vi "Curtin1_Acquire.vi"(8 "MainVI":refnum<vi>, 11 "Settings":T3={"Name of test"="ScratchPad", "Date"=timestamp(0 s since 1904-01-01), "Location"="Home", "Template"="ScratchPad", "Soundcard"="OCTA-CAPTURE", "resolution"=32, "Sampling rate"=48000, "Ch1 Gain "=25.0, "Ch2 Gain"=10.0, "Sample time (s)"=0.3, "Pre-trigger (s)"=0.001, "Hammer Threshold"=10.0, "Positions"=12, "Taps/Position"=5, "Set Names"="H,V", "Freq resolution"=1.0, "Hammer cutoff"=0.025, "Mic cutoff"=0.25, "Double bounce "=10.0, "Hammer Cal"=10.0, "dB Offset"=0.0, "Accel Cal"=10.0, "Vibrometer Cal"=0.0, "Mic Cal"=0.0, "Output"=2, "Voltage Cal"=0.01, "Vibrometer Port"="ASRL27::INSTR", "Range"=4, "High Pass"=2, "Bandwidth"=4, "X Range"=[], "Y Range"=[], "dB Spread"=0.0, "Trigger"=0, "Ch_1"=25, "Ch_2"=25, "flip?"=FALSE, "60Hz"=FALSE, "Time offset"=0.0, "Piezo Cal"=1.0, "Default Notes"="", "Tom"=FALSE} {"Ch_2" min=1 step=1; "Ch_1" min=1 max=100 step=1; "Trigger" items=["Hammer (force)", "Self-tap", "Spacebar"]; "Bandwidth" items=["1 kHz"=1, "5 kHz"=5, "10 kHz"=10, "25 kHz"=25, "50 kHz"=50, "100 kHz"=100]; "High Pass" items=["Off", "13 Hz", "104 Hz"]; "Range" items=["10 mm/s"=1, "20 mm/s"=2, "50 mm/s"=5, "100 mm/s"=10, "200 mm/s"=20, "500 mm/s"=50, "1 m/s"=100, "2 m/s"=200]; "Output" items=["Accelerometer", "Speed (from acceleration)", "Microphone", "Vibrometer", "Piezo"]; "Voltage Cal" format="%#_13g"; "Ch2 Gain" format="%#_13g"; "Ch1 Gain" format="%#_13g"; "Double bounce" min=0.0; "Mic cutoff" min=0.0 format="%#_4g"; "Hammer cutoff" min=0.0 format="%#_4g"; "Freq resolution" min=0.0; "Pre-trigger (s)" format="%#_13g"; "Date" format="%<%H:%M\n%d/%m/%y>T"; "resolution" items=["16 bit"=16, "24 bit"=24, "32 bit"=32]; "Sampling rate" items=["22050 samp/s"=22050, "44100 samp/s"=44100, "48000 samp/s"=48000]}) -> (1 "Name Change?":bool, 2 "Data?":bool, 3 "Average FRF":cluster{dbl, "df":dbl, dbl[]}[](graph))   [LabVIEW 2022 SP3]
uses:
  <extravilib>/ChannelInstances/Tag-a[.](wfm(dbl)).lvlib
  Mic/Mic_Global.vi
  <extravilib>/ChannelInstances/Lossy Stream-a[.](wfm(dbl)).lvlib
  AmpCtrl.ctl
  PreferencesControl.ctl
panel:
  in  "Record Button":bool=TRUE
  in  "Tab Control":enum32{"graphs", "settings", "Notes"}(tab)
  in  "AddPhoto":bool
  out "color":string
  in  "Move":bool
  in  "Motor Settings":bool
  in  "Tap":bool
  in  "Method":enum16{"Sqrt(H1H2)", "H1", "H2"}(ring)
  in  "History":bool=TRUE
  in  "Help":bool
  in  "Beam":bool
  in  "rescale Y Axes":bool
  in  "Open Sound":bool
  in  "View":u16(ring) items=["Raw", "Volts", "Units (Pa, N, etc)"]
  out "Hammer Spectrum":cluster{dbl, "df":dbl, "FFT {X}":dbl[]}[](graph)
  out "Hammer Data":cluster{dbl, "dt":dbl, "Y":dbl[]}[](graph)
  out "Microphone Data":cluster{dbl, "dt":dbl, "Y":dbl[]}[](graph)
  out "Volume":T1 {"Mic" scale=0.0..100.0; "Hammer" scale=0.0..100.0}
  in  "OpenVibrometer":bool
  in  "New":bool
  in  "Save SP":bool
  in  "Export":bool
  in  "Plot View":T2={"Alerts"=FALSE, "Log X Axis"=TRUE, "dB scale"=TRUE, "Averaging"=TRUE, "Fade"=0.0, "Centroids?"=FALSE, "line thickness"=1}
  in  "Locked":bool
  in  "Notes":string
  in  "Done":bool
  out "Progress Bar":picture
  in  "zoom":bool
  in  "dB Spread":dbl=40.0
  in  "rescale Y":bool
  in  "stop":bool
  out "Alarms":string
  in  "Colors":u16(ring) items=["24 Colors", "rear"]
  # "Hz"
  # "dB"
  # "dB"
  # "sec"
  # "sec"
  # "mV/Pa"
  # "mV/m/s2"
  # "mV/mm/s"
  # "V/N"
  # "sec"
  # "sec"
  # "mV/N"
  # "%"
  # "%"
  # "sec"
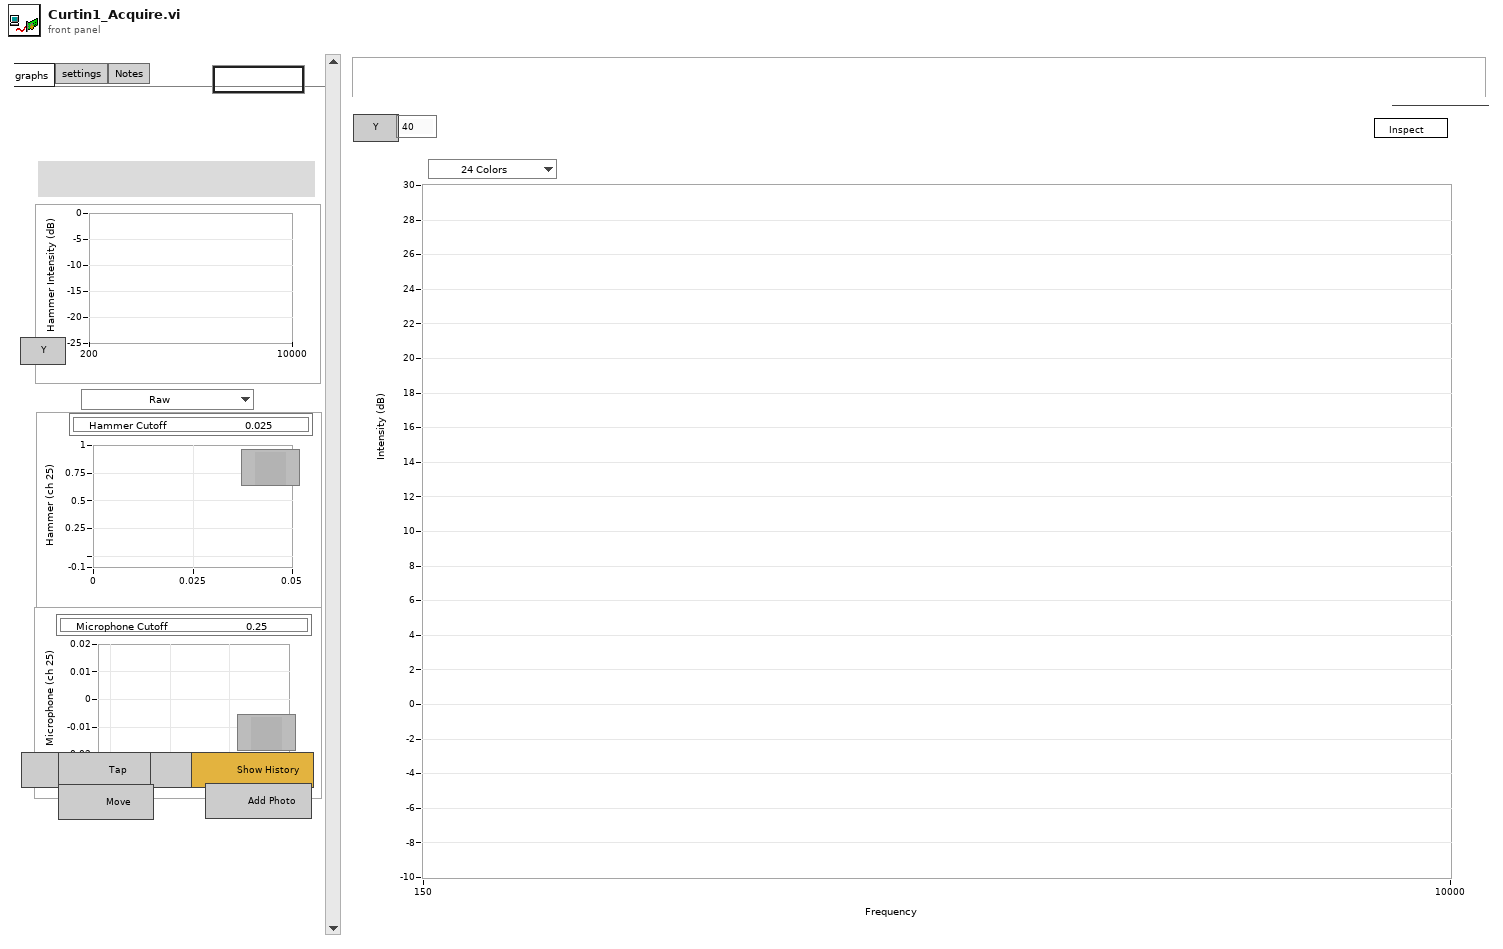
[diagram p1: front panel]
types:
  T1 = typedef "AmpCtrl.ctl" = cluster{"Hammer":u8, "Mic":u8, "Mic In":string}
  T2 = cluster{"Alerts":bool, "Log X Axis":bool, "dB scale":bool, "Averaging":bool, "Fade":dbl, "Centroids?":bool, "line thickness":u8}
  T3 = typedef "PreferencesControl.ctl" = cluster{"Name of test":string, "Date":timestamp, "Location":string, "Template":string, "Soundcard":string, "resolution":u16, "Sampling rate":u16, "Ch1 Gain ":dbl, "Ch2 Gain":dbl, "Sample time (s)":dbl, "Pre-trigger (s)":dbl, "Hammer Threshold":dbl, "Positions":i16, "Taps/Position":i16, "Set Names":string, "Freq resolution":dbl, "Hammer cutoff":dbl, "Mic cutoff":dbl, "Double bounce ":dbl, "Hammer Cal":dbl, "dB Offset":dbl, "Accel Cal":dbl, "Vibrometer Cal":dbl, "Mic Cal":dbl, "Output":u16, "Voltage Cal":dbl, "Vibrometer Port":refnum<visa-resource-name>, "Range":u16, "High Pass":u16, "Bandwidth":u16, "X Range":cluster{"Minimum":dbl, "Maximum":dbl, "Increment":dbl, "Minor Increment":dbl, "Start":dbl}[], "Y Range":cluster{"Minimum":dbl, "Maximum":dbl, "Increment":dbl, "Minor Increment":dbl, "Start":dbl}[], "dB Spread":dbl, "Trigger":u16, "Ch_1":u8, "Ch_2":u8, "flip?":bool, "60Hz":bool, "Time offset":dbl, "Piezo Cal":dbl, "Default Notes":string, "Tom":bool}
  T4 = enum32{"Invalid", "Standard", "Closed", "Hidden", "Minimized", "Maximized"}
  T5 = enum16{"Initialize", "Free run", "One Shot - waiting", "One Shot - triggered", "Wait", "Close"}
  T6 = enum16{"Always On", "Always Off", "Off While Running"}
  T7 = enum8{"Enabled", "Disabled", "Disabled and Grayed Out"}
  T8 = typedef "Tag-a[.](wfm(dbl)).lvlib/))Channel.ctl" = refnum<queue>
  T9 = typedef "Lossy Stream-a[.](wfm(dbl)).lvlib/)Channel.ctl" = refnum<queue>
  T10 = typedef "LVBoundsTypeDef.ctl" = cluster{"Width":u32, "Height":u32}
  T11 = cluster{"Minimum":dbl, "Maximum":dbl, "Increment":dbl, "Minor Increment":dbl, "Start":dbl}
  T12 = typedef "eventvkey.ctl" = enum16{"ASCII", "Enter", "Return", "Shift", "Ctrl", "Alt", "Cmd", "Opt", "Caps", "NumLock", "Clear", "Break", "Up", "Down", "Left", "Right", "Insert", "Delete", "Home", "End", "PageUp", "PageDown", "Escape", "Help", "Pause", "ScrollLock", "F1", "F2", "F3", "F4", "F5", "F6", "F7", "F8", "F9", "F10", "F11", "F12", "F13", "F14", "F15", "F16", "F17", "F18", "F19", "F20", "F21", "F22", "F23", "F24", "Play", "VolumeUp", "VolumeDown", "Mute", "Two Byte Char"}
  T13 = typedef "LVMouseTypeDef.ctl" = cluster{"Mouse Position":cluster{"X":i32, "Y":i32}, "Mouse Modifiers":cluster{"Button Down":bool, "Shift Mod":bool, "Menu Mod":bool, "Option Mod":bool}}
  T14 = typedef "LVRangeTypeDef.ctl" = cluster{"Minimum":dbl, "Maximum":dbl, "Increment":dbl, "Minor Increment":dbl, "Start":dbl}
  T15 = cluster{"Minimum":dbl, "Maximum":dbl, "Increment":dbl, "Minor Increment":dbl, "Start":dbl}[]
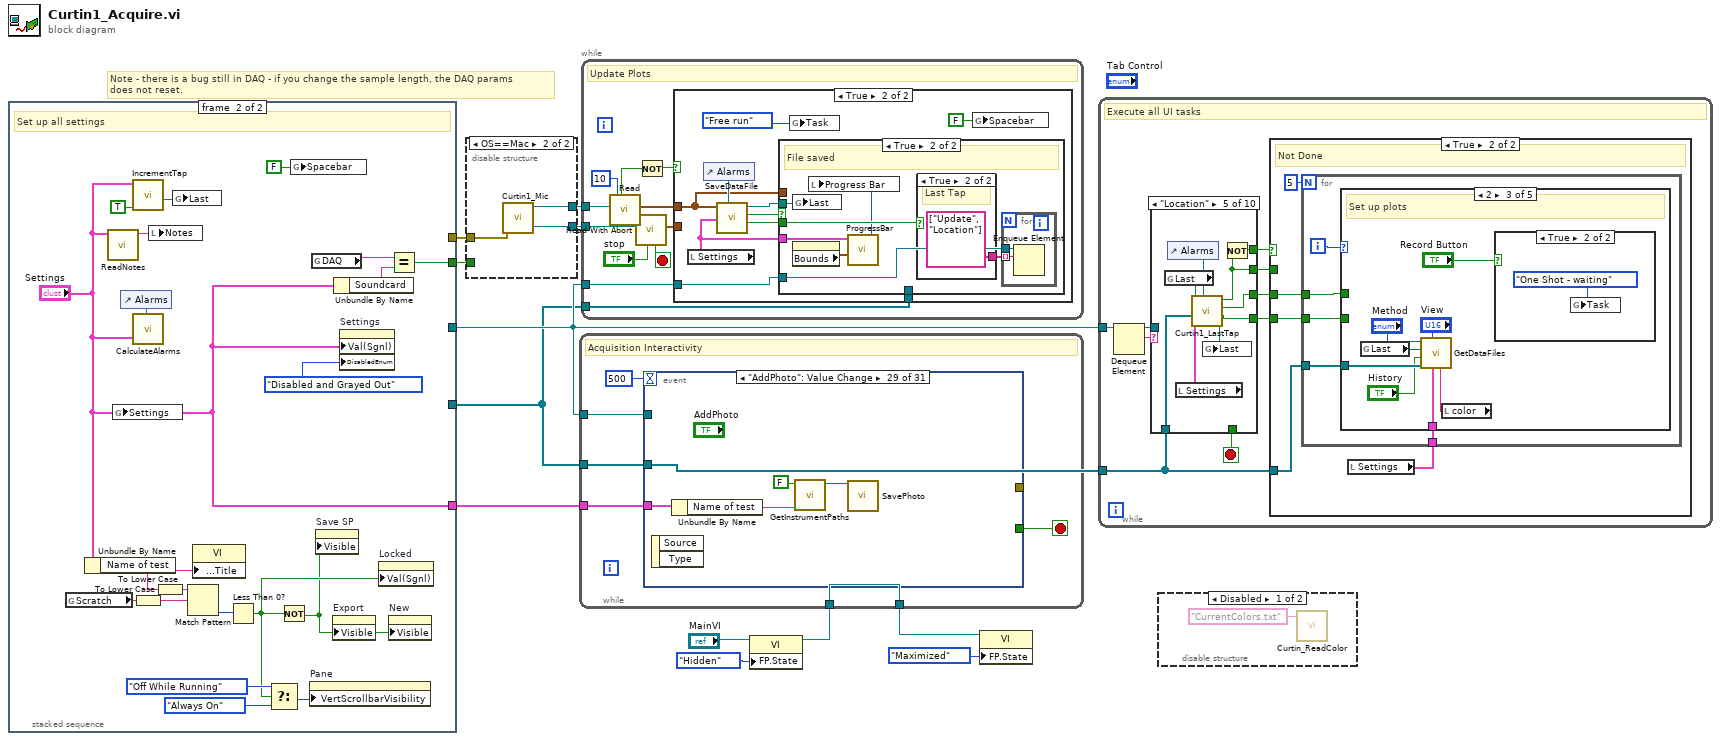
[diagram p0: block diagram]
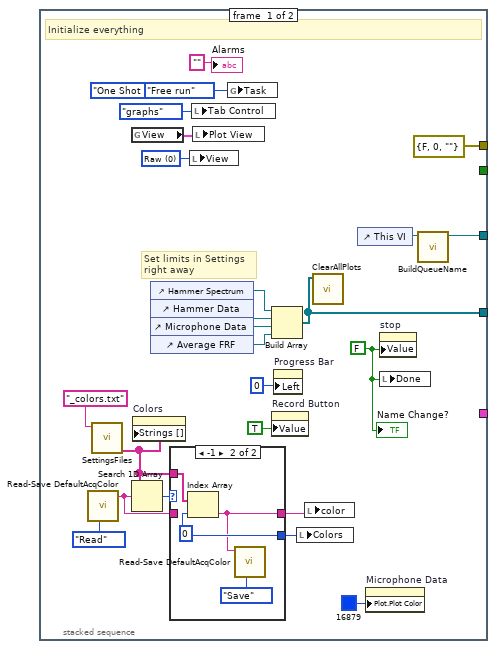
[diagram p3: hidden frame]
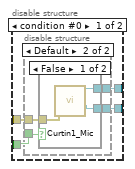
[diagram p5: hidden frame]
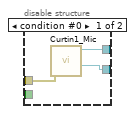
[diagram p6: hidden frame]
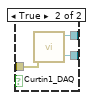
[diagram p7: hidden frame]
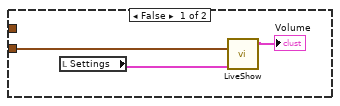
[diagram p8: hidden frame]
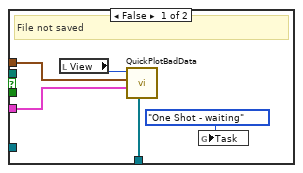
[diagram p9: hidden frame]
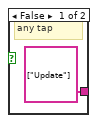
[diagram p10: hidden frame]
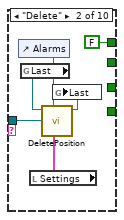
[diagram p12: hidden frame]
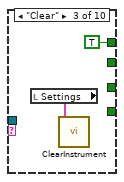
[diagram p13: hidden frame]
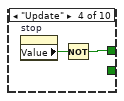
[diagram p14: hidden frame]
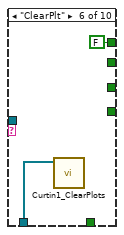
[diagram p15: hidden frame]
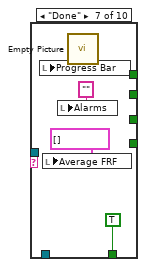
[diagram p16: hidden frame]
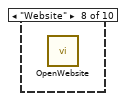
[diagram p17: hidden frame]
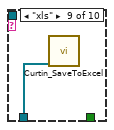
[diagram p18: hidden frame]
diagram:
  # "Note - there is a bug still in DAQ - if you change the sample length, the DAQ params \ndoes not reset."
  n1 = stacked-sequence {
    tunnel: [_ "Settings"] -> w5
    tunnel: [_ w52] -> w4
    tunnel: [w26 _] -> w3
    tunnel: [errorcluster {"status"=FALSE, "code"=0, "source"=""} ("error in (no error)") _] -> w2
    tunnel: [w20 _] -> w1
    frame #0 {
      w33 = u16 0 items=["Raw", "Volts", "Units (Pa, N, etc)"] ("View")
      w35 = FALSE ("stop")
      # "Set limits in Settings \nright away"
      # "Initialize everything"
      n2 = call "Read-Save DefaultAcqColor.vi"("Task"=enum16{"Save", "Read"}."Read") -> ("palette name Out"=w13:string)  [unwired: 9 in, 1 out]
      n3 = call "SettingsFiles.vi"("settings file name"="_colors.txt" ("pattern")) -> ("filenames"=w14:string[])  [unwired: 9 in, 1 out]
      n4 = global read "Mic_Global.vi" "View"() -> (w36:T2)
      n5 = Search 1D Array(1D array=w14, element=w13) -> (index of element=w15:i32)  [unwired: 1 in]
      n6 = property on="Colors" class="Ring (strict)"("Strings []"=w14) -> ()  [unwired: 2 in, 2 out]
      n7 = control-ref of="Hammer Spectrum"() -> (w21:refnum<vi>)
      n8 = control-ref of="Hammer Data"() -> (w22:refnum<vi>)
      n9 = control-ref of="Microphone Data"() -> (w23:refnum<vi>)
      n10 = control-ref of="Average FRF"() -> (w24:refnum<vi>)
      n11 = case shown="-1" w15 {
        selector: w15 -> [w38 _]
        tunnel: [w38 w43] -> w18
        tunnel: [w39 w40] -> w17
        tunnel: w14 -> [_ w42]
        tunnel: w13 -> [w39 _]
        frame Default {
        }
        frame -1 {
          w43 = 0
          n12 = Index Array(array=w42, index=w43) -> (element=w40:string)
          n13 = call "Read-Save DefaultAcqColor.vi"("Task"=enum16{"Save", "Read"}."Save", "acq color palette"=w40) -> ()  [unwired: 8 in, 2 out]
        }
      }
      n14 = local write "View"(w33) -> ()
      n15 = local write "Tab Control"(enum32{"graphs", "settings"}."graphs" ("Tab Control")) -> ()
      n16 = local write "Plot View"(w36) -> ()
      n17 = global write "Mic_Global.vi" "Task"(T5."One Shot - waiting" ("Task")) -> ()
      n18 = global write "Mic_Global.vi" "Task"(T5."Free run" ("Task")) -> ()
      n19 = Build Array(w21, w22, w23, w24) -> (w20:refnum<vi>[])
      n20 = property on="Record Button" class="Bool (strict)"("Value"=TRUE ("Good point?")) -> ()  [unwired: 2 in, 2 out]
      n21 = property on="Progress Bar" class="Pict"("Left"=i16 0 ("Origin:Left")) -> ()  [unwired: 2 in, 2 out]
      n22 = local write "Colors"(w18) -> ()
      n23 = local write "color"(w17) -> ()
      n24 = call "ClearAllPlots.vi"("Array"=w20) -> ()  [unwired: 11 in]
      n25 = control-ref of="This VI"() -> (w27:refnum<vi>)
      n26 = property on="Microphone Data" class="WFGraph (strict)"("Plot.Plot Color"=u32 16879) -> ()  [unwired: 2 in, 2 out]
      n27 = property on="stop" class="Bool (strict)"("Value"=w35) -> ()  [unwired: 2 in, 2 out]
      n28 = local write "Done"(w35) -> ()
      n29 = call "BuildQueueName.vi"("VI in"=w27) -> ("Queue out"=w26:refnum<queue>)  [unwired: 9 in, 1 out]
      "Name Change?" <- w35
      "Alarms" <- "" ("Alarms")
    }
    frame #1 {
      # "Set up all settings"
      n30 = global read "Mic_Global.vi" "Scratch"() -> (w58:string)
      n31 = Unbundle By Name("Settings") -> ("Name of test"=w57:string)
      n32 = call "ReadNotes.vi"("Settings"="Settings") -> ("Notes"=w62:string)  [unwired: 9 in, 1 out]
      n33 = global write "Mic_Global.vi" "Settings"("Settings") -> ()
      n34 = control-ref of="Alarms"() -> (w59:refnum<vi>)
      n35 = call "IncrementTap.vi"("Reset?"=TRUE, "Settings"="Settings") -> ("Last Data Set"=w61:path)  [unwired: 4 in, 5 out]
      n36 = call "CalculateAlarms.vi"("Settings"="Settings", "Alarm"=w59) -> ()  [unwired: 8 in, 2 out]
      n37 = To Lower Case(string=w58) -> (all lower case string=w45:string)
      n38 = local write "Notes"(w62) -> ()
      n39 = To Lower Case(string=w57) -> (all lower case string=w46:string)
      n40 = global write "Mic_Global.vi" "Last"(w61) -> ()
      n41 = Match Pattern(string=w46, regular expression=w45) -> (offset past match=w56:i32)  [unwired: 1 in, 3 out]
      n42 = property class="VI"("Front Panel.Title"=w57) -> ()  [unwired: 2 in, 2 out]
      n43 = Less Than 0?(x=w56) -> (x < 0?=w48:bool)
      n44 = Select(t=T6."Off While Running" ("Vertical Scrollbar Visibility"), s=w48, f=T6."Always On" ("Vertical Scrollbar Visibility")) -> (s? t:f=w55:T6)
      n45 = Not(x=w48) -> (.not. x?=w47:bool)
      n46 = global write "Mic_Global.vi" "Spacebar"(FALSE ("Spacebar")) -> ()
      n47 = property on="Pane" class="Pane"("VertScrollbarVisibility"=w55) -> ()  [unwired: 2 in, 2 out]
      n48 = global read "Mic_Global.vi" "DAQ"() -> (w54:string)
      n49 = property on="Save SP" class="Bool"("Visible"=w47) -> ()  [unwired: 2 in, 2 out]
      n50 = property on="Export" class="Bool"("Visible"=w47) -> ()  [unwired: 2 in, 2 out]
      n51 = Unbundle By Name("Settings") -> ("Soundcard"=w53:string)
      n52 = property on="Settings" class="Clust (strict)"("Val(Sgnl)"="Settings", "DisabledEnum"=T7."Disabled and Grayed Out" ("Disabled")) -> ()  [unwired: 2 in, 2 out]
      n53 = property on="Locked" class="Bool (strict)"("Val(Sgnl)"=w48) -> ()  [unwired: 2 in, 2 out]
      n54 = Equal?(x=w54, y=w53) -> (x = y?=w52:bool)
      n55 = property on="New" class="Bool"("Visible"=w47) -> ()  [unwired: 2 in, 2 out]
    }
  }
  n56 = disable-structure shown="OS==Mac" {
    disable-tunnel: w2 -> [w67 w83]
    disable-tunnel: [w66 w81] -> w12
    disable-tunnel: [w65 w82] -> w11
    disable-tunnel: w4 -> [w64 _]
    frame condition #0 {
      n57 = disable-structure shown="Default" {
        disable-tunnel: w67 -> [w68 w72]
        disable-tunnel: [w70 w74] -> w66
        disable-tunnel: [w69 w73] -> w65
        disable-tunnel: w64 -> [_ w71]
        frame condition #0 {
          n58 = call "Curtin1_Mic.vi"("error in (no error)"=w68) -> ("latest data"=w70:T8, "Tap"=w69:T9)  [unwired: 9 in]
        }
        frame condition #1 (active) {
          n59 = case shown="False" w71 {
            tunnel: [w76 w80] -> w74
            tunnel: [w75 w79] -> w73
            tunnel: w72 -> [w77 w78]
            frame False {
              n60 = call "Curtin1_Mic.vi"("error in (no error)"=w77) -> ("latest data"=w76:T8, "Tap"=w75:T9)  [unwired: 9 in]
            }
            frame True {
              n61 = call "Curtin1_DAQ.vi"("error in (no error)"=w78) -> ("Buffer"=w80:T8, "Tap"=w79:T9)  [unwired: 9 in]
            }
          }
        }
      }
    }
    frame condition #1 (active) {
      n62 = call "Curtin1_Mic.vi"("error in (no error)"=w83) -> ("latest data"=w81:T8, "Tap"=w82:T9)  [unwired: 9 in]
    }
  }
  n63 = while {
    tunnel: w11 -> [w94]
    tunnel: w12 -> [w91]
    tunnel: w3 -> [w85]
    tunnel: w1 -> [w84]
    stop <- w90 stop-if-true
    # "Update Plots"
    n64 = call <extravilib>:"Read.vi"("channel"=w94, "timeout in ms (-1)"=10) -> ("element"=w93:waveform(dbl)[], "timed out?"=w87:bool)  [unwired: 4 in, 4 out]
    n65 = call <extravilib>:"Read With Abort.vi"("abort"="stop", "channel"=w91) -> ("element"=w89:waveform(dbl)[], "aborted?"=w90:bool)  [unwired: 7 in, 1 out]
    n66 = Not(x=w87) -> (.not. x?=w86:bool)
    n67 = case shown="True" w86 {
      tunnel: w93 -> [_ w100]
      tunnel: w89 -> [w96 _]
      tunnel: w85 -> [_ w105]
      tunnel: w84 -> [_ w99]
      frame False {
        n68 = local read "Settings"() -> (w95:T3)
        n69 = call "LiveShow.vi"("Settings"=w95, "Buffer"=w96) -> ("Volume"=→"Volume":T1)  [unwired: 9 in]
      }
      frame True {
        n70 = local read "Settings"() -> (w101:T3)
        n71 = control-ref of="Alarms"() -> (w104:refnum<vi>)
        n72 = call "SaveDataFile.vi"("Settings"=w101, "Alarms"=w104, "Data"=w100) -> ("last tap?"=w106:bool, "New File?"=w107:bool, "new path"=w103:path)  [unwired: 4 in, 2 out]
        n73 = case shown="True" w107 {
          tunnel: w106 -> [_ w119]
          tunnel: w105 -> [_ w113]
          tunnel: w103 -> [_ w118]
          tunnel: w101 -> [w108 w116]
          tunnel: w100 -> [w109 _]
          tunnel: w99 -> [w110 _]
          frame False {
            # "File not saved"
            n74 = local read "View"() -> (w111:u16)
            n75 = call "QuickPlotBadData.vi"("Array"=w110, "Settings"=w108, "Data"=w109, "View"=w111) -> ()  [unwired: 8 in]
            n76 = global write "Mic_Global.vi" "Task"(T5."One Shot - waiting" ("Task")) -> ()
          }
          frame True {
            # "File saved"
            n77 = global write "Mic_Global.vi" "Last"(w118) -> ()
            n78 = property on="Progress Bar" class="Pict"() -> ("Bounds"=w114:T10)  [unwired: 2 in, 2 out]
            n79 = call "ProgressBar.vi"("Bounds"=w114, "Settings"=w116) -> ("Progress Bar"=w115:picture)  [unwired: 7 in, 2 out]
            n80 = local write "Progress Bar"(w115) -> ()
            n81 = case shown="True" w119 {
              tunnel: [string[] ["Update"] string[] ["Update", "Location"]] -> w117
              frame False {
                # "any tap"
              }
              frame True {
                # "Last Tap"
              }
            }
            n82 = for {
              tunnel: w117 -> [w121] mode=indexing
              tunnel: w113 -> [w120]
              n83 = Enqueue Element(queue=w120, element=w121) -> ()  [unwired: 2 in, 3 out]
            }
          }
        }
        n84 = global write "Mic_Global.vi" "Task"(T5."Free run" ("Task")) -> ()
        n85 = global write "Mic_Global.vi" "Spacebar"(FALSE ("Spacebar")) -> ()
      }
    }
  }
  n86 = property class="VI"(reference="MainVI", "FP.State"=T4."Hidden" ("Front Panel Window:State")) -> (reference out=w6:refnum<vi>)  [unwired: 1 in, 1 out]
  n87 = while {
    tunnel: w1 -> [w129]
    tunnel: w3 -> [w126]
    tunnel: [w125] -> w7
    tunnel: w6 -> [w125]
    tunnel: w5 -> [w124]
    stop <- w127 stop-if-true
    # "Acquisition Interactivity"
    n88 = event shown="[28] \"AddPhoto\": Value Change" {
      selector: _ -> [_ _ _ _ _ _ _ _ _ _ _ _ _ _ _ _ _ _ _ _ _ _ _ _ _ _ _ _ _ _ _]
      dyn-events: _ -> [_ _ _ _ _ _ _ _ _ _ _ _ _ _ _ _ _ _ _ _ _ _ _ _ _ _ _ _ _ _ _]
      timeout: 500 -> [_ _ _ _ _ _ _ _ _ _ _ _ _ _ _ _ _ _ _ _ _ _ _ _ _ _ _ _ _ _ _]
      tunnel: [_ _ _ _ _ _ _ _ _ _ _ _ _ _ _ _ _ _ _ w263 _ _ _ _ _ _ _ _ _ _ w304] -> w127
      tunnel: w129 -> [w133 w145 _ _ _ w164 _ _ _ _ _ _ _ w209 _ _ _ _ _ _ _ _ _ _ _ _ _ _ _ _ _]
      tunnel: w126 -> [_ _ _ _ _ w168 _ w174 w179 w193 w200 w203 _ w208 _ _ _ _ _ w262 _ w278 _ _ _ _ _ _ _ _ w303]
      tunnel: [_ _ _ _ _ _ _ _ _ _ _ _ _ _ _ _ _ _ w248 _ _ _ _ _ _ w289 w295 _ _ _ _] -> _
      tunnel: w124 -> [_ _ _ _ _ _ _ _ _ _ _ _ _ _ _ _ w238 _ _ w258 _ _ _ w285 _ w288 _ _ w300 _ _]
      event "Hammer Data", "Microphone Data", "Average FRF", "Hammer Spectrum": Mouse Up {
        n89 = event-data() -> ("PlatMods.Shift"=w134:bool, "CtlRef"=w132:refnum<vi>)  [unwired: 1 in]
        n90 = local read "History"() -> (w136:bool)
        n91 = Search 1D Array(1D array=w133, element=w132) -> (index of element=w131:i32)  [unwired: 1 in]
        n92 = case shown="1, 2" w131 {
          tunnel: [9 0] -> w130
          frame 1, 2 {
          }
          frame Default {
          }
        }
        n93 = call "BuildZoomNames.vi"("History"=w136, "WaveformGraph in"=w132) -> ("Names"=w135:string[])  [unwired: 9 in]
        n94 = case shown="True" w134 {
          tunnel: w132 -> [_ w142]
          tunnel: w135 -> [_ w140]
          tunnel: w130 -> [_ w139]
          frame False {
          }
          frame True {
            n95 = local read "dB Spread"() -> (w141:dbl)
            n96 = call "GraphZoom.vi"("Plot"=w139, "Names"=w140, "dB Range"=w141, "Graph"=w142) -> ()  [unwired: 8 in]
          }
        }
      }
      event "zoom": Value Change {
        n97 = event-data() -> ()  [unwired: 1 in, 1 out]
        n98 = Index Array(array=w145, index=3) -> (element=w143:refnum<vi>)
        n99 = local read "History"() -> (w148:bool)
        n100 = call "BuildZoomNames.vi"("History"=w148, "WaveformGraph in"=w143) -> ("Names"=w147:string[])  [unwired: 9 in]
        n101 = local read "dB Spread"() -> (w146:dbl)
        n102 = call "GraphZoom.vi"("Names"=w147, "dB Range"=w146, "Graph"=w143) -> ()  [unwired: 9 in]
      }
      event "Microphone Data": Cursor Move {
        n103 = event-data() -> ("CursLoc.X"=w149:dbl)  [unwired: 1 in]
        n104 = property on="Mic cutoff" class="DigNum (strict)"("Val(Sgnl)"=w149) -> ()  [unwired: 2 in, 2 out]
      }
      event "Hammer Data": Cursor Move {
        n105 = event-data() -> ("CursIdx"=w151:i32, "CursLoc.X"=w152:dbl, "CursLoc.Y"=w150:dbl)  [unwired: 1 in]
        n106 = case shown="0" w151 {
          tunnel: w152 -> [w153 _]
          tunnel: w150 -> [_ w154]
          frame 0 {
            n107 = property on="Hammer cutoff" class="DigNum (strict)"("Val(Sgnl)"=w153) -> ()  [unwired: 2 in, 2 out]
          }
          frame Default {
            n108 = property on="Hammer Threshold" class="DigNum (strict)"("Val(Sgnl)"=w154) -> ()  [unwired: 2 in, 2 out]
          }
        }
      }
      event "Notes": Value Change {
        n109 = event-data() -> ()  [unwired: 1 in, 1 out]
        n110 = local read "Settings"() -> (w156:T3)
        n111 = call "Curtin1_SaveNotesFile.vi"("Notes"="Notes", "Settings in"=w156) -> ()  [unwired: 10 in]
      }
      event Value Change {
        n112 = event-data() -> ("NewVal"=w162:T3, "OldVal"=w161:T3)  [unwired: 1 in]
        n113 = Enqueue Element(queue=w168, element="Update") -> ()  [unwired: 2 in, 3 out]
        n114 = call "VibrometerSettings.vi"("OldVal"=w161, "NewVal"=w162) -> ("Settings"=w157:T3)  [unwired: 5 in, 4 out]
        n115 = global write "Mic_Global.vi" "Settings"(w157) -> ()
        n116 = call "Curtin1_SaveLastSettingsFile.vi"("Settings in"=w157) -> ()  [unwired: 11 in]
        n117 = call "Curtin1_updatePlots.vi"("plots"=w164, "Settings"=w157) -> ()  [unwired: 10 in]
        n118 = Unbundle By Name(w157) -> ("dB Spread"=w163:dbl, "Output"=w159:u16)
        n119 = call "Read_Write_Test_Parameters.vi"("Task"=enum16{"Save", "Read", "Clear"}."Save", "Settings"=w157) -> ("Settings"=w165:T3)  [unwired: 8 in, 1 out]
        n120 = local write "dB Spread"(w163) -> ()
        n121 = call "IncrementTap.vi"("Settings"=w165) -> ("Last Data Set"=w166:path)  [unwired: 5 in, 5 out]
        n122 = Equal?(x=u16 3 ("Output"), y=w159) -> (x = y?=w158:bool)
        n123 = global write "Mic_Global.vi" "Last"(w166) -> ()
        n124 = property on="Beam" class="Bool (strict)"("Visible"=w158) -> ()  [unwired: 2 in, 2 out]
      }
      event "dB Spread": Value Change {
        n125 = event-data() -> ("NewVal"=w171:dbl)  [unwired: 1 in]
        n126 = local read "Settings"() -> (w172:T3)
        n127 = Bundle By Name(cluster=w172, "dB Spread"=w171) -> (w170:T3)
        n128 = local write "Settings"(w170) -> ()
        n129 = global write "Mic_Global.vi" "Settings"(w170) -> ()
      }
      event Key Up {
        n130 = event-data() -> ("ScanCode"=w176:i16, "PlatMods.Shift"=w175:bool)  [unwired: 1 in]
        n131 = call "Check KeyUp.vi"("Shift"=w175, "ScanCode"=w176) -> ("Task"=w173:string)  [unwired: 9 in]
        n132 = case shown="Default" w173 {
          selector: w173 -> [_ w177]
          tunnel: w174 -> [_ w178]
          frame "" {
          }
          frame Default {
            n133 = Enqueue Element(queue=w178, element=w177) -> ()  [unwired: 2 in, 3 out]
          }
        }
      }
      event Key Down {
        n134 = event-data() -> ("VKey"=w180:T12)  [unwired: 1 in, 3 out]
        n135 = case shown="\"Up\", \"Down\"" w180 {
          selector: w180 -> [_ w184 w188]
          tunnel: w179 -> [_ w181 w186]
          frame "ASCII", Default {
          }
          frame "Left", "Right" {
            n136 = Format Into String(w184) -> (resulting string=w183:string)  [unwired: 3 in, 1 out]
            n137 = Enqueue Element(queue=w181, element="Update") -> ()  [unwired: 2 in, 3 out]
            n138 = call "FadeLeftRight.vi"("Key"=w183) -> ()  [unwired: 11 in]
          }
          frame "Up", "Down" {
            n139 = Format Into String(w188) -> (resulting string=w185:string)  [unwired: 3 in, 1 out]
            n140 = Enqueue Element(queue=w186, element="Update") -> ()  [unwired: 2 in, 3 out]
            n141 = call "ThicknessUpDown.vi"("Key"=w185) -> ()  [unwired: 11 in]
          }
        }
      }
      event "Progress Bar": Mouse Up {
        # "need to end free run\nif in Done condition"
        n142 = event-data() -> ()  [unwired: 1 in, 1 out]
        n143 = property on="Progress Bar" class="Pict"() -> ("Mouse"=w194:T13, "Bounds"=w192:T10)  [unwired: 2 in, 2 out]
        n144 = local read "Settings"() -> (w191:T3)
        n145 = global write "Mic_Global.vi" "Task"(T5."Free run" ("Task")) -> ()
        n146 = call "DetermineSetChosen.vi"("Settings"=w191, "Bounds"=w192, "Mouse"=w194) -> ("Queue Task"=w189:string)  [unwired: 7 in, 1 out]
        n147 = case shown="Default" w189 {
          selector: w189 -> [_ w195]
          tunnel: w193 -> [_ w198]
          tunnel: w191 -> [_ w197]
          frame "" {
          }
          frame Default {
            n148 = Enqueue Element(queue=w198, element=w195) -> ()  [unwired: 2 in, 3 out]
            n149 = control-ref of="Alarms"() -> (w196:refnum<vi>)
            n150 = call "CalculateAlarms.vi"("Settings"=w197, "Alarm"=w196) -> ()  [unwired: 8 in, 2 out]
          }
        }
      }
      event "Plot View": Value Change {
        n151 = event-data() -> ()  [unwired: 1 in, 4 out]
        n152 = Enqueue Element(queue=w200, element="Update") -> ()  [unwired: 2 in, 3 out]
        n153 = global write "Mic_Global.vi" "View"("Plot View") -> ()
      }
      event "View", "History", "Method": Value Change {
        n154 = event-data() -> ()  [unwired: 1 in, 4 out]
        n155 = Enqueue Element(queue=w203, element="Update") -> ()  [unwired: 2 in, 3 out]
      }
      event "Record Button": Value Change {
        n156 = event-data() -> ("NewVal"=w204:bool)  [unwired: 1 in]
        n157 = Select(t=T5."One Shot - waiting" ("Task"), s=w204, f=T5."Free run" ("Task")) -> (s? t:f=w206:T5)
        n158 = global write "Mic_Global.vi" "Task"(w206) -> ()
      }
      event "Average FRF", "Hammer Spectrum", "Microphone Data", "Hammer Data": Scale Range Change; "rescale Y": Value Change {
        n159 = event-data() -> ()  [unwired: 1 in, 1 out]
        n160 = stacked-sequence {
          tunnel: w209 -> [w211 w222 _]
          tunnel: w208 -> [_ _ w223]
          frame #0 {
            n161 = case shown="False" "rescale Y" {
              tunnel: w211 -> [_ w217]
              tunnel: "dB Spread" -> [_ w214]
              frame False {
              }
              frame True {
                n162 = Index Array(array=w217, index=3) -> (element=w215:refnum<vi>)
                n163 = call "AutoscaleYaxis.vi"("Has Coherence in plot?"=TRUE, "dB Range"=w214, "WaveformGraph in"=w215) -> ()  [unwired: 9 in]
              }
            }
          }
          frame #1 {
            n164 = call "GetPlotRanges.vi"("plots"=w222) -> ("Yscales"=w219:T14[], "Xscales"=w220:T14[])  [unwired: 9 in]
            n165 = local read "Settings"() -> (w221:T3)
            n166 = Bundle By Name(cluster=w221, "X Range"=w220, "Y Range"=w219) -> (w218:T3)
            n167 = property on="Settings" class="Clust (strict)"("Val(Sgnl)"=w218) -> ()  [unwired: 2 in, 2 out]
          }
          frame #2 {
            # "done in settings update"
            n168 = disable-structure shown="Disabled" {
              disable-tunnel: w223 -> [w224 _]
              frame Disabled {
                n169 = Enqueue Element(queue=w224, element="Update") -> ()  [unwired: 2 in, 3 out]
              }
              frame Enabled {
              }
            }
          }
        }
      }
      event "Locked": Value Change {
        n170 = event-data() -> ()  [unwired: 1 in, 1 out]
        n171 = property on="Export" class="Bool"() -> ("Visible"=w229:bool)  [unwired: 2 in, 2 out]
        n172 = Not(x=w229) -> (.not. x?=w228:bool)
        n173 = Not(x="Locked") -> (.not. x?=w226:bool)
        n174 = Select(t=T7."Disabled and Grayed Out" ("Disabled"), s="Locked", f=T7."Enabled" ("Disabled")) -> (s? t:f=w232:T7)
        n175 = And(x=w226, y=w228) -> (x .and. y?=w227:bool)
        n176 = property on="Settings" class="Clust (strict)"("DisabledEnum"=w232) -> ()  [unwired: 2 in, 2 out]
        n177 = property on="Save SP" class="Bool"("Visible"=w226) -> ()  [unwired: 2 in, 2 out]
        n178 = case shown="True" w227 {
          tunnel: "Warning: You should not edit these parameters in the middle of a run.  Instead, play around in ScratchPad and then Export your new settings as a template." -> [_ w235]
          frame False {
          }
          frame True {
            n179 = One Button Dialog(message=w235) -> ()  [unwired: 1 in, 1 out]
          }
        }
      }
      event "Export": Value Change {
        n180 = event-data() -> ()  [unwired: 1 in, 3 out]
        n181 = local read "Settings"() -> (w236:T3)
        n182 = call "Curtin_SaveTemplate.vi"("Settings in"=w236) -> ()  [unwired: 8 in, 3 out]
      }
      event "Save SP": Value Change {
        n183 = event-data() -> ()  [unwired: 1 in, 1 out]
        n184 = local read "Settings"() -> (w239:T3)
        n185 = call "CheckForTemplateEdits.vi"("Original Settings"=w238, "Force?"=TRUE, "Current Settings"=w239) -> ()  [unwired: 8 in, 1 out]
      }
      event "New": Value Change {
        n186 = event-data() -> ()  [unwired: 1 in, 3 out]
        n187 = local read "Settings"() -> (w244:T3)
        n188 = local write "Name Change?"(TRUE ("Name Change?")) -> ()
        n189 = property on="Record Button" class="Bool (strict)"("Value"=FALSE ("Good point?")) -> ()  [unwired: 2 in, 2 out]
        n190 = call "RenameScratchtoTest.vi"("Settings"=w244) -> ("Ok?"=w245:bool, "Name of test"=w242:string, "Settings Out"=w241:T3)  [unwired: 8 in]
        n191 = case shown="True" w245 {
          tunnel: w242 -> [_ w247]
          tunnel: w241 -> [_ w246]
          frame False {
          }
          frame True {
            n192 = local write "Settings"(w246) -> ()
            n193 = global write "Mic_Global.vi" "Settings"(w246) -> ()
            n194 = property class="VI"("Front Panel.Title"=w247) -> ()  [unwired: 2 in, 2 out]
          }
        }
      }
      event "Open Sound": Value Change {
        # "F1 will open this"
        n195 = event-data() -> ()  [unwired: 1 in, 3 out]
        n196 = Open VI Reference(vi path="Curtin1_Mic.vi") -> (vi reference=w251:refnum<vi>, error out=w249:errorcluster)  [unwired: 5 in]
        n197 = invoke class="VI" method="FP.Open"(reference=w251, error in=w249, "Activate"=TRUE ("Activate?")) -> (error out=w248:errorcluster)  [unwired: 2 in, 4 out]
      }
      event "stop": Value Change {
        w260 = cluster{dbl, "df":dbl, dbl[]}[] [] ("Average FRF")
        # "Do not ask if you only changed axis ranges"
        n198 = event-data() -> ("NewVal"=w263:bool)  [unwired: 1 in]
        n199 = call "Read_Write_Test_Parameters.vi"("Task"=enum16{"Save", "Read", "Clear"}."Read", "Settings"=w258) -> ("Settings"=w257:T3)  [unwired: 8 in, 1 out]
        n200 = local read "Settings"() -> (w255:T3)
        n201 = Enqueue Element(queue=w262, element="Done") -> ()  [unwired: 2 in, 3 out]
        n202 = call "CheckForTemplateEdits.vi"("Original Settings"=w257, "Force?"=FALSE, "Current Settings"=w255) -> ("Current Settings out"=w253:T3)  [unwired: 8 in]
        n203 = global write "Mic_Global.vi" "Settings"(w255) -> ()
        n204 = call "CheckScratchAndExit.vi"("Settings"=w253) -> ("Ask?"=→"Data?":bool)  [unwired: 10 in]
        "Microphone Data" <- w260
        "Hammer Data" <- w260
        "Hammer Spectrum" <- w260
        "Average FRF" <- w260
      }
      event "rescale Y Axes": Value Change {
        n205 = event-data() -> ()  [unwired: 1 in, 1 out]
        n206 = local read "Settings"() -> (w265:T3)
        n207 = Unbundle By Name(w265) -> ("Y Range"=w264:T15, "Trigger"=w266:u16)
        n208 = case shown="0, Default" w266 {
          tunnel: w265 -> [w273 _]
          tunnel: w264 -> [w268 _]
          frame 0, Default {
            n209 = Replace Array Subset(array=w268, new element #1=T11 {"Minimum"=-0.1, "Maximum"=1.0, "Increment"=0.2, "Minor Increment"=0.05, "Start"=0.0} ("XScale.Range"), index #1=1 ("index"), new element #2=T11 {"Minimum"=-1.0, "Maximum"=1.0, "Increment"=0.5, "Minor Increment"=0.1, "Start"=-1.0} ("XScale.Range")) -> (w267:T15)  [unwired: 1 in]
            n210 = Bundle By Name(cluster=w273, "Y Range"=w267) -> (w272:T3)
            n211 = property on="Settings" class="Clust (strict)"("Val(Sgnl)"=w272) -> ()  [unwired: 2 in, 2 out]
          }
          frame 1 {
            w274 = u8 1 ("Y Scale.Scale Fit")
            n212 = property on="Hammer Data" class="WFGraph (strict)"("YScale.ScaleFit"=w274) -> ()  [unwired: 2 in, 2 out]
            n213 = property on="Microphone Data" class="WFGraph (strict)"("YScale.ScaleFit"=w274) -> ()  [unwired: 2 in, 2 out]
          }
        }
      }
      event "Colors": Value Change {
        n214 = event-data() -> ()  [unwired: 1 in, 2 out]
        n215 = Enqueue Element(queue=w278, element="Update") -> ()  [unwired: 2 in, 3 out]
        n216 = property on="Colors" class="Ring (strict)"() -> ("Strings []"=w279:string[], "Value"=w280:u16)  [unwired: 2 in, 2 out]
        n217 = Index Array(array=w279, index=w280) -> (element=w275:string)
        "color" <- w275
        n218 = call "Read-Save DefaultAcqColor.vi"("Task"=enum16{"Save", "Read"}."Save", "acq color palette"=w275) -> ()  [unwired: 8 in, 2 out]
      }
      event "Beam": Value Change {
        n219 = event-data() -> ()  [unwired: 1 in, 2 out]
        n220 = local read "Settings"() -> (w283:T3)
        n221 = Unbundle By Name(w283) -> ("Vibrometer Port"=w282:refnum<visa-resource-name>)
        n222 = call "Toggle Laser.vi"("Beam"="Beam", "RS232"=w282) -> ()  [unwired: 8 in, 2 out]
      }
      event "OpenVibrometer": Value Change {
        n223 = event-data() -> ()  [unwired: 1 in, 2 out]
        n224 = call "PolyTec_Control_Panel.vi"("Settings in"=w285) -> ("Settings Out"=w284:T3)  [unwired: 8 in, 2 out]
        n225 = property on="Settings" class="Clust (strict)"("Val(Sgnl)"=w284) -> ()  [unwired: 2 in, 2 out]
      }
      event "Motor Settings": Value Change {
        n226 = event-data() -> ()  [unwired: 1 in, 2 out]
        n227 = case shown="True" "Motor Settings" {
          frame False {
          }
          frame True {
            n228 = call "MotorControl.vi"() -> ()  [unwired: 12 in]
          }
        }
      }
      event "Tap": Value Change {
        n229 = event-data() -> ()  [unwired: 1 in, 2 out]
        n230 = Unbundle By Name(w288) -> ("Taps/Position"=w287:i16)
        n231 = for {
          N: w287 -> [_]
          tunnel: [w292] -> w289
          n232 = call "Motor_OpenSendRead.vi"("Angle to move"=-1) -> ("error out"=w292:errorcluster)  [unwired: 8 in, 2 out]
          n233 = Wait (ms)(milliseconds to wait=u32 1000) -> ()  [unwired: 1 out]
        }
      }
      event "Move": Value Change {
        n234 = event-data() -> ()  [unwired: 1 in, 2 out]
        n235 = local read "Settings"() -> (w294:T3)
        n236 = call "Automation Control.vi"("Settings"=w294) -> ("desired position"=w293:dbl)  [unwired: 10 in]
        n237 = call "Motor_OpenSendRead.vi"("Angle to move"=w293) -> ("error out"=w295:errorcluster)  [unwired: 8 in, 2 out]
      }
      event "Help": Value Change {
        n238 = event-data() -> ()  [unwired: 1 in, 2 out]
        n239 = One Button Dialog(message="Hints:\n1. Cutoffs: Move the green lines to zero out noise data (replace acquired data with zero for all future times)\n2. Hammer trigger (purple line) lets you choose how hard the hammer has to hit to trigger a dataset\n3. click on Notes (at top) to add thoughts ") -> ()  [unwired: 1 in, 1 out]
      }
      event "AddPhoto": Value Change {
        n240 = event-data() -> ()  [unwired: 1 in, 2 out]
        n241 = Unbundle By Name(w300) -> ("Name of test"=w297:string)
        n242 = call "GetInstrumentPaths.vi"("Instrument"=w297, "Build?"=FALSE) -> ("Path To Instrument Folder"=w298:path)  [unwired: 5 in, 4 out]
        n243 = call "SavePhoto.vi"("Instrument path"=w298) -> ()  [unwired: 10 in, 1 out]
      }
      event Panel Close? {
        n244 = event-data() -> ()  [unwired: 1 in, 1 out]
        n245 = property on="stop" class="Bool (strict)"("Val(Sgnl)"=TRUE ("Value (Signaling)")) -> ()  [unwired: 2 in, 2 out]
        n246 = event-data("Discard?"=TRUE) -> ()  [unwired: 1 in, 1 out]
      }
      event Timeout {
        n247 = event-data() -> ()  [unwired: 1 in, 1 out]
        n248 = case shown="True" "Done" {
          tunnel: [_ w308] -> w304
          tunnel: w303 -> [_ w307]
          frame False {
          }
          frame True {
            w308 = TRUE ("Value (Signaling)")
            n249 = Enqueue Element(queue=w307, element="Done") -> ()  [unwired: 2 in, 3 out]
            n250 = property on="stop" class="Bool (strict)"("Value"=w308) -> ()  [unwired: 2 in, 2 out]
          }
        }
      }
    }
  }
  n251 = property class="VI"(reference=w7, "FP.State"=T4."Maximized" ("Front Panel Window:State")) -> ()  [unwired: 1 in, 2 out]
  n252 = while {
    tunnel: w1 -> [w314]
    tunnel: w3 -> [w315]
    stop <- w316 stop-if-true
    # "Execute all UI tasks"
    n253 = Dequeue Element(queue=w315) -> (queue out=w310:refnum<queue>, element=w313:string)  [unwired: 2 in, 2 out]
    n254 = case shown="\"Location\"" w313 {
      tunnel: [_ FALSE TRUE w326 w332 FALSE _ _ _ _] -> w317
      tunnel: [_ _ _ _ _ _ TRUE _ _ _] -> w316
      tunnel: w314 -> [_ _ _ _ w336 w337 _ _ w343 _]
      tunnel: [_ _ _ _ w331 _ _ _ _ _] -> w312
      tunnel: [_ _ _ _ w329 _ _ _ _ _] -> w311
      tunnel: w310 -> [_ w320 _ _ _ _ _ _ _ _]
      tunnel: [_ _ _ _ w328 _ _ _ _ _] -> w309
      frame Default {
      }
      frame "Delete" {
        n255 = control-ref of="Alarms"() -> (w319:refnum<vi>)
        n256 = global read "Mic_Global.vi" "Last"() -> (w322:path)
        n257 = local read "Settings"() -> (w318:T3)
        n258 = call "DeletePosition.vi"("Settings"=w318, "Alarms"=w319, "queue"=w320, "last"=w322) -> ("Last Data Set"=w321:path)  [unwired: 6 in, 1 out]
        n259 = global write "Mic_Global.vi" "Last"(w321) -> ()
      }
      frame "Clear" {
        n260 = local read "Settings"() -> (w324:T3)
        n261 = call "ClearInstrument.vi"("Settings"=w324) -> ()  [unwired: 11 in]
      }
      frame "Update" {
        n262 = property on="stop" class="Bool (strict)"() -> ("Value"=w327:bool)  [unwired: 2 in, 2 out]
        n263 = Not(x=w327) -> (.not. x?=w326:bool)
      }
      frame "Location" {
        n264 = global read "Mic_Global.vi" "Last"() -> (w335:path)
        n265 = control-ref of="Alarms"() -> (w330:refnum<vi>)
        n266 = local read "Settings"() -> (w334:T3)
        n267 = call "Curtin1_LastTap.vi"("Alarms"=w330, "Plots"=w336, "Settings"=w334, "Data"=w335) -> ("Data Out"=w333:path, "New Set"=w331:bool, "Pause?"=w329:bool, "Done?"=w328:bool)  [unwired: 4 in]
        n268 = global write "Mic_Global.vi" "Last"(w333) -> ()
        n269 = Not(x=w328) -> (.not. x?=w332:bool)
      }
      frame "ClearPlt" {
        n270 = call "Curtin1_ClearPlots.vi"("Array"=w337) -> ()  [unwired: 11 in]
      }
      frame "Done" {
        n271 = local write "Average FRF"(cluster{dbl, "df":dbl, dbl[]}[] [] ("Average FRF")) -> ()
        n272 = local write "Alarms"("") -> ()
        n273 = call "Empty Picture"() -> ("empty picture"=w341:picture)
        n274 = local write "Progress Bar"(w341) -> ()
      }
      frame "Website" {
        n275 = call "OpenWebsite.vi"() -> ()  [unwired: 12 in]
      }
      frame "xls" {
        n276 = call "Curtin_SaveToExcel.vi"("plots"=w343) -> ()  [unwired: 11 in]
      }
      frame "Close" {
      }
    }
    n277 = case shown="True" w317 {
      tunnel: w314 -> [_ w349]
      tunnel: w312 -> [_ w348]
      tunnel: w311 -> [_ w347]
      tunnel: w309 -> [w344 _]
      frame False {
        # "Dont refresh"
        n278 = case shown="False" w344 {
          frame False {
          }
          frame True {
            n279 = property on="stop" class="Bool (strict)"("Val(Sgnl)"=TRUE ("Value (Signaling)")) -> ()  [unwired: 2 in, 2 out]
          }
        }
      }
      frame True {
        # "Not Done"
        n280 = local read "Settings"() -> (w346:T3)
        n281 = for {
          N: 5 ("timeout in ms (-1)") -> [_]
          tunnel: w349 -> [w354]
          tunnel: w348 -> [w353]
          tunnel: w347 -> [w352]
          tunnel: w346 -> [w351]
          i -> [w355]
          n282 = case shown="2" w355 {
            tunnel: w354 -> [_ _ w373 _ _]
            tunnel: w351 -> [_ w361 w371 w375 _]
            tunnel: w353 -> [_ _ _ _ _]
            tunnel: w352 -> [w356 _ _ _ _]
            frame 0 {
              # "Check fo Pause"
              n283 = case shown="True" w356 {
                frame False {
                }
                frame True {
                  n284 = property on="Record Button" class="Bool (strict)"("Val(Sgnl)"=FALSE ("Record Button")) -> ()  [unwired: 2 in, 2 out]
                }
              }
            }
            frame 1 {
              # "set cursors positions"
              n285 = Unbundle By Name(w361) -> ("Hammer cutoff"=w365:dbl, "Mic cutoff"=w364:dbl)
              n286 = call "Curtin1_SoundCardCorrection.vi"("Settings"=w361) -> ("Converted"=w359:dbl[])  [unwired: 5 in, 5 out]
              n287 = local read "View"() -> (w360:u16)
              n288 = Index Array(array=w359, index=w360) -> (element=w358:dbl)
              n289 = property on="Hammer Data" class="WFGraph (strict)"("Active Cursor"=u32 0, "Cursor.Cursor X"=w365) -> ()  [unwired: 2 in, 2 out]
              n290 = property on="Microphone Data" class="WFGraph (strict)"("Cursor.Cursor X"=w364) -> ()  [unwired: 2 in, 2 out]
              n291 = property on="Hammer Data" class="WFGraph (strict)"("Active Cursor"=u32 1, "Cursor.Cursor Y"=w358) -> ()  [unwired: 2 in, 2 out]
            }
            frame 2 {
              # "Set up plots"
              n292 = global read "Mic_Global.vi" "Last"() -> (w370:path)
              n293 = local read "color"() -> (w366:string)
              n294 = call "GetDataFiles.vi"("Color scheme"=w366, "Settings"=w371, "View"="View", "plots"=w373, "Show history"="History", "path"=w370, "Method"="Method") -> ()  [unwired: 5 out]
              n295 = case shown="True" "Record Button" {
                frame False {
                }
                frame True {
                  n296 = global write "Mic_Global.vi" "Task"(T5."One Shot - waiting" ("Task")) -> ()
                }
              }
            }
            frame 3 {
              # "Check for last point and redraw progress"
              n297 = property on="Progress Bar" class="Pict"() -> ("Bounds"=w376:T10)  [unwired: 2 in, 2 out]
              n298 = call "ProgressBar.vi"("Bounds"=w376, "Settings"=w375) -> ("Progress Bar"=→"Progress Bar":picture)  [unwired: 7 in, 2 out]
            }
            frame Default {
            }
          }
        }
      }
    }
  }
  n299 = disable-structure shown="Disabled" {
    frame Disabled {
      n300 = call "Curtin_ReadColor.vi"("color file name"="CurrentColors.txt" ("name or relative path")) -> ()  [unwired: 1 in, 2 out]
    }
    frame Enabled {
    }
  }
